vi "Read All Dictionary Elements.vi"(8 "error in (no error)":errorcluster, 11 "Control Experiment":refnum<class "Control Experiment.lvclass">) -> (0 "error out":errorcluster, 2 "items":T1[](array[typedef]), 3 "Control Experiment out":refnum<class "Control Experiment.lvclass">)   [LabVIEW 2019, in "Control Experiment.lvclass"]
uses:
  Control Experiment.lvclass
  <userlib>/LevyLab/LV-Data/LV-Data/Typedefs/Dictionary--cluster.ctl
  <userlib>/LevyLab/LV-Data/LV-Data/LV-Data.lvclass
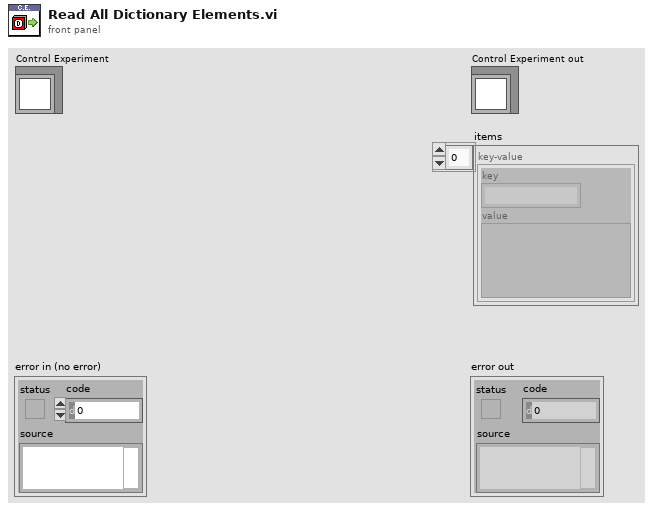
[diagram p1: front panel]
types:
  T1 = typedef "LV-Data.lvclass/Dictionary--cluster.ctl" = cluster{"key":string, "value":variant}
  T2 = typedef "Dictionary Object RefNum__ogtk.ctl" = refnum<k1>
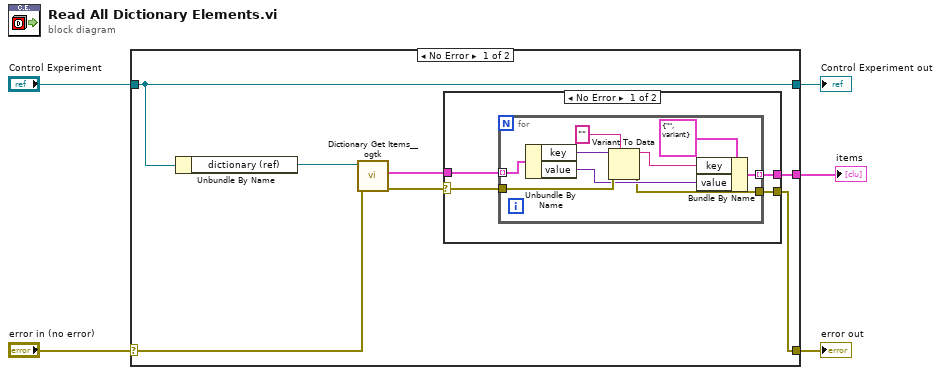
[diagram p0: block diagram]
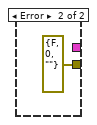
[diagram p2: hidden frame]
diagram:
  n1 = case shown="No Error" "error in (no error)" {
    selector: "error in (no error)" -> [w10 w27]
    tunnel: [w6 w27] -> w4
    tunnel: [w12 w28] -> w2
    tunnel: "Control Experiment" -> [w12 w28]
    tunnel: [w8 _] -> w1
    frame No Error {
      n2 = Unbundle By Name(w12) -> ("dictionary (ref)"=w11:T2)
      n3 = call <userlib>:"Dictionary Get Items__ogtk.vi"("error in (no error)"=w10, "dictionary"=w11) -> ("error out"=w7:errorcluster, "items"=w9:cluster{"key":variant, "value":variant}[])  [unwired: 7 in, 1 out]
      n4 = case shown="No Error" w7 {
        selector: w7 -> [w14 _]
        tunnel: w9 -> [w16 _]
        tunnel: [w15 _] -> w8
        tunnel: [w13 errorcluster {"status"=FALSE, "code"=0, "source"=""} ("error out")] -> w6
        frame No Error {
          n5 = for {
            tunnel: w16 -> [w24] mode=indexing
            tunnel: [w25] -> w15 mode=indexing
            tunnel: w14 -> [w20]
            tunnel: [w18] -> w13
            n6 = Unbundle By Name(w24) -> ("key"=w23:variant, "value"=w19:variant)
            n7 = Variant To Data(error in=w20, type="" ("key"), Variant=w23) -> (data=w21:string, error out=w18:errorcluster)
            n8 = Bundle By Name(cluster=T1 {"key"="", "value"=variant} ("key-value"), "key"=w21, "value"=w19) -> (w25:T1)
          }
        }
        frame Error {
        }
      }
    }
    frame Error {
    }
  }
  "error out" <- w4
  "Control Experiment out" <- w2
  "items" <- w1
